vi "Main.vi"() -> ()   [LabVIEW 2020]
uses:
  Global Variables/Global Number of Indices.vi
  Global Variables/Training_Status.vi
  Global Variables/Number_of_Windows.vi
  Global Variables/Window_Size.vi
  Global Variables/Global Label.vi
  Global Variables/Global N-Back Setting.vi
  Global Variables/Trainning Done.vi
  Global Variables/Global Send To ANN.vi
  Global Variables/Global Difficulty Level.vi
  Global Variables/Global Enable Logging.vi
  Global Variables/Global User_Answer.vi
  Global Variables/Global Correct Answer.vi
panel:
  out "Difficulty Level":u8
  out "tiggerTime":u32
  out "New square":T1
  out "seq":i8
  out "Data":bool[](array[boolean])
  out "error out":errorcluster
  out "2D Picture":picture
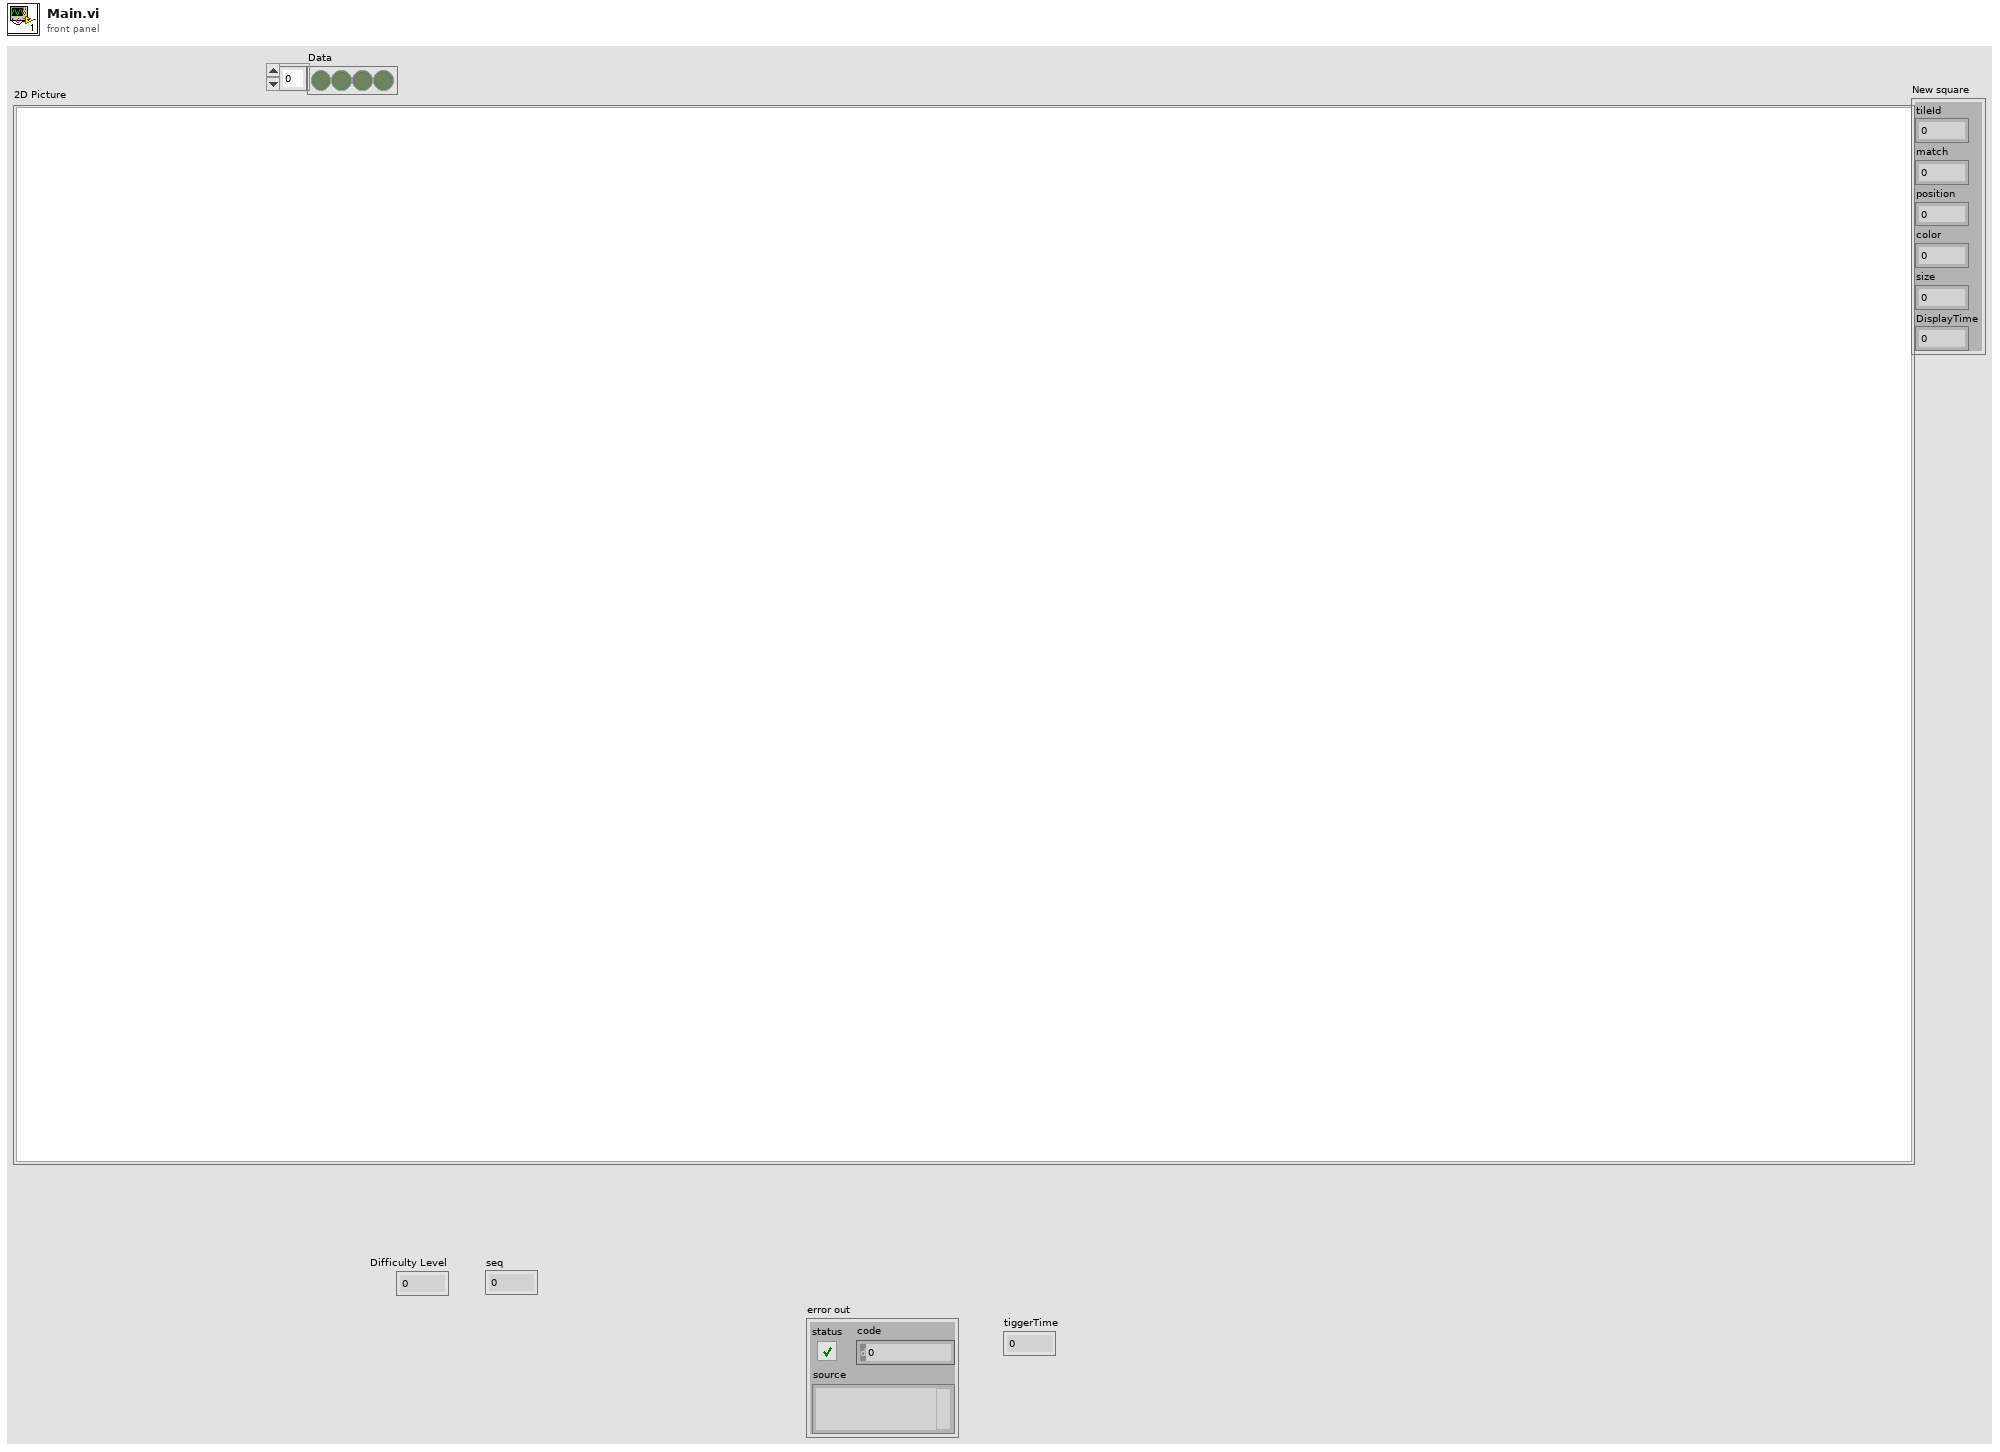
[diagram p1: front panel]
types:
  T1 = cluster{"tileId":i32, "match":i32, "position":i32, "color":u32, "size":i32, "DisplayTime":i32}
  T2 = cluster{"State":i32, "Iteration":i8, "Sequence":i8, "Counter":i8}
  T3 = cluster{"Tile size Y":dbl, "Columns":dbl, "Rows":dbl, "Cross size":dbl, "Offset X":dbl, "Tile size X":dbl, "OffsetY":dbl}
  T4 = cluster{"tileId":i32, "match":i32, "position":i32, "color":u32, "size":i32, "DisplayTime":i32}[]
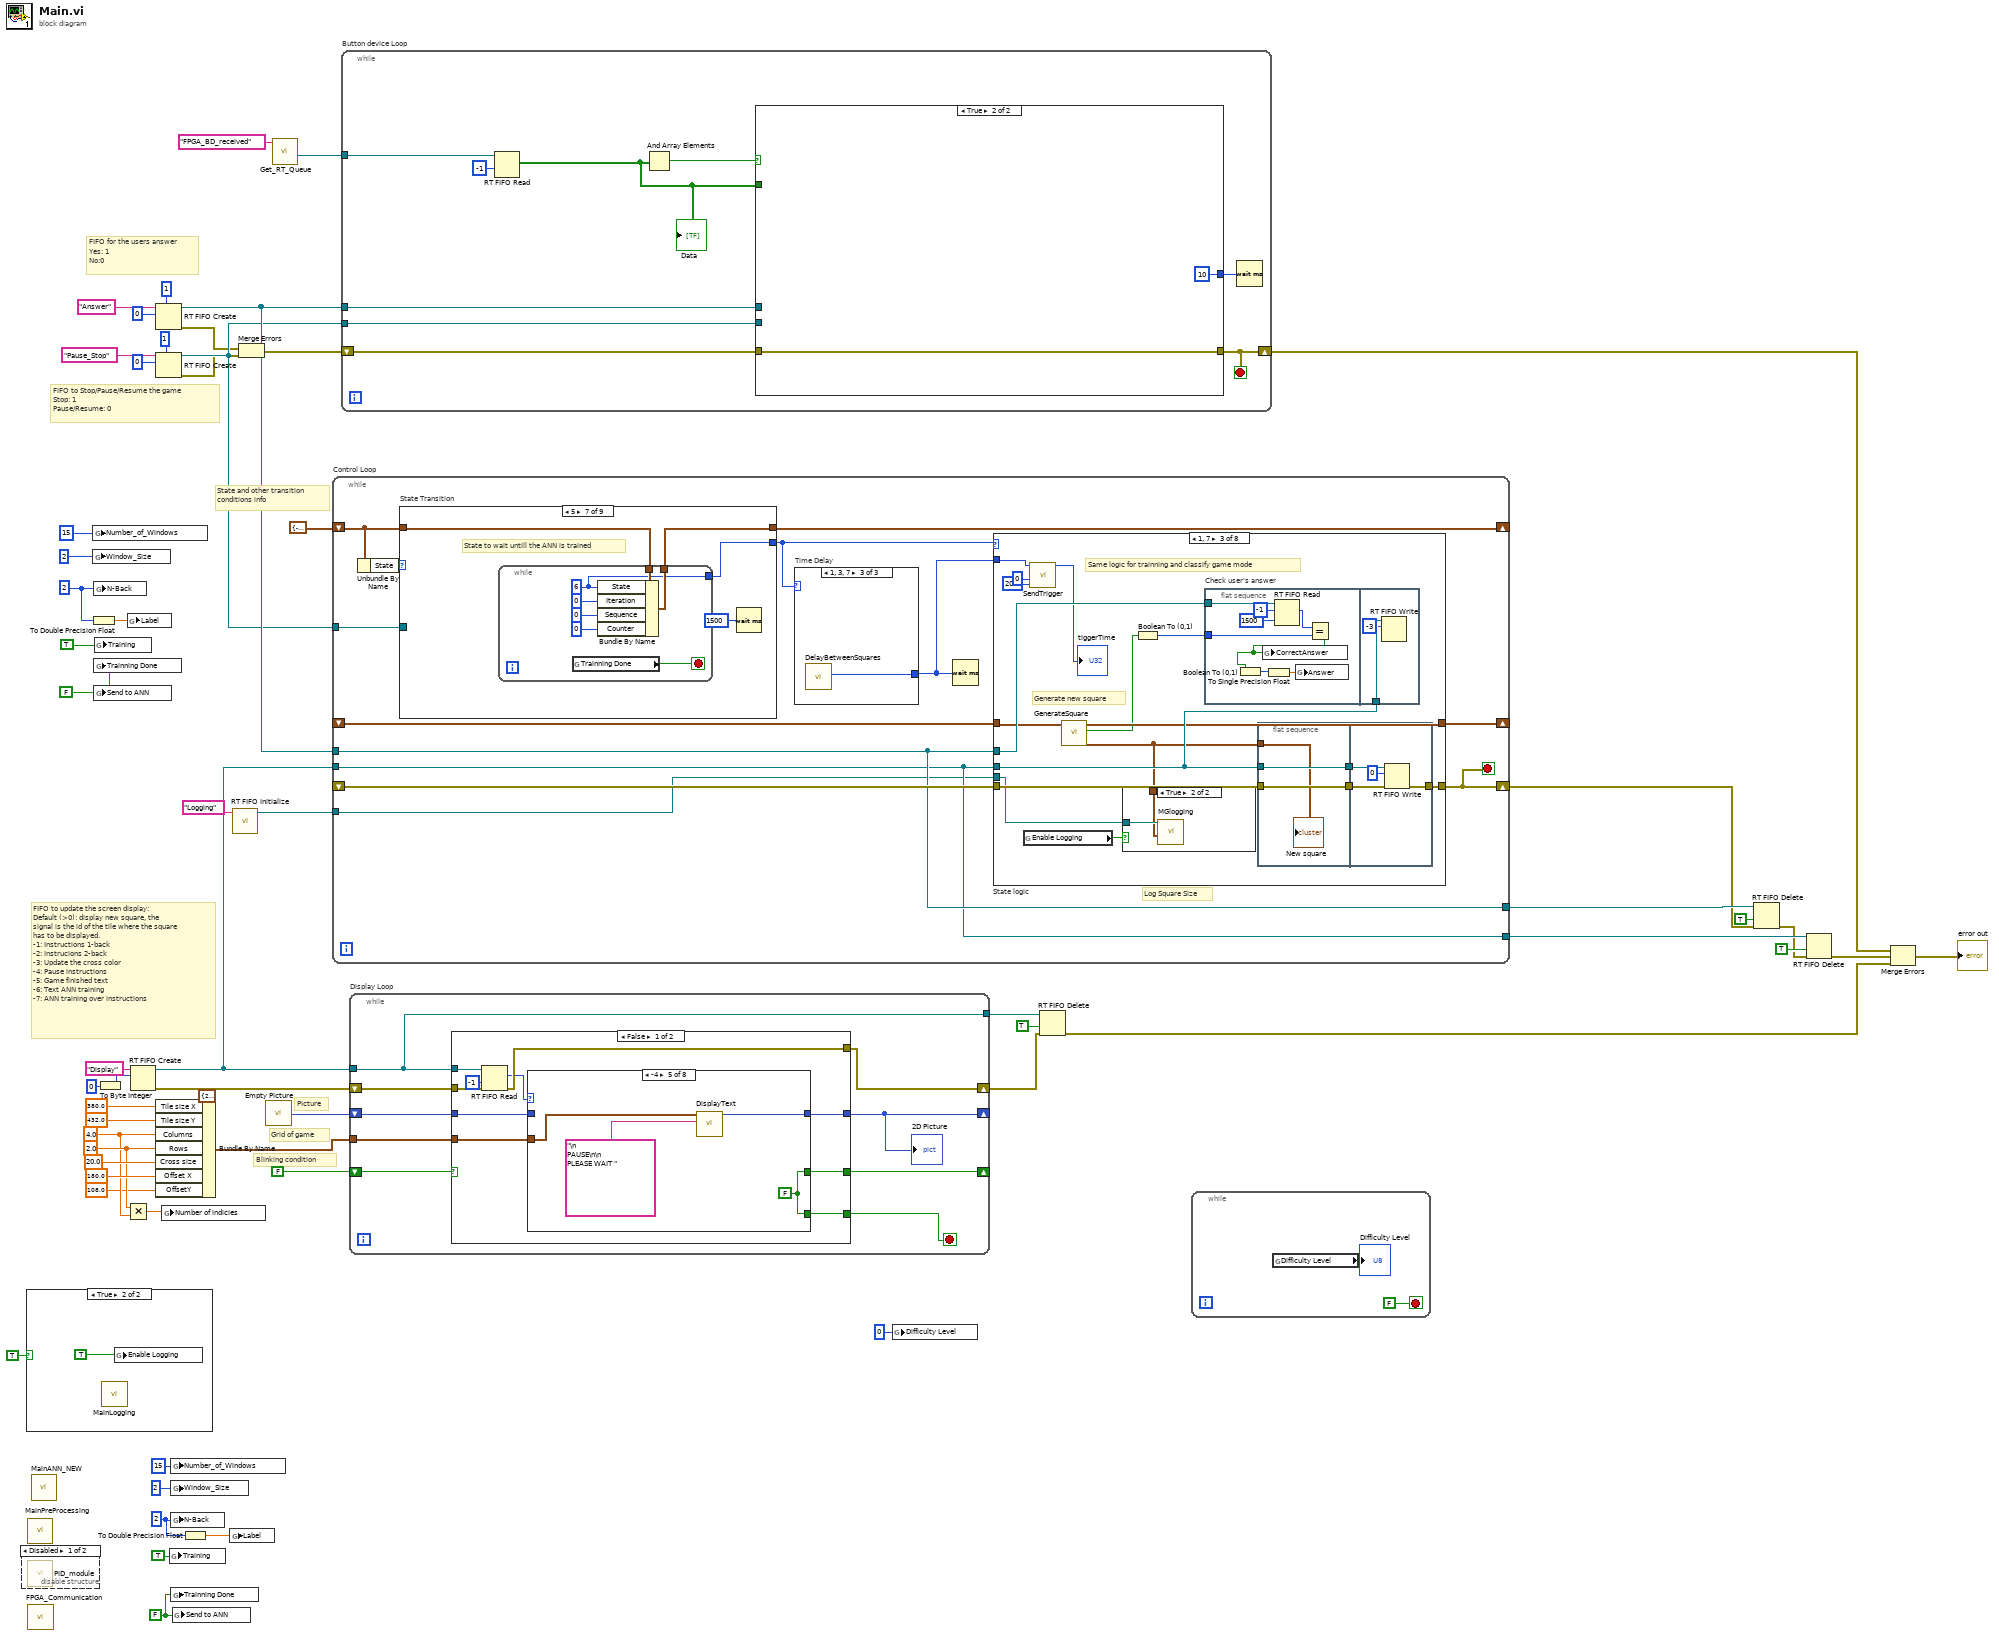
[diagram p0: block diagram]
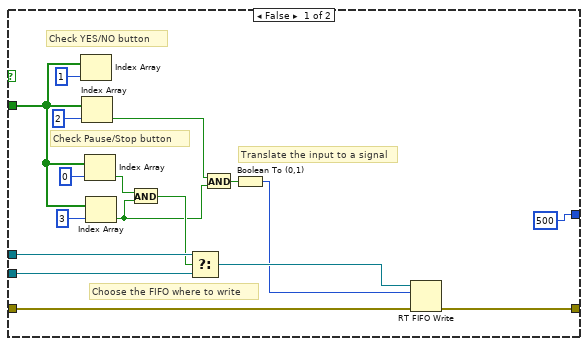
[diagram p3: hidden frame]
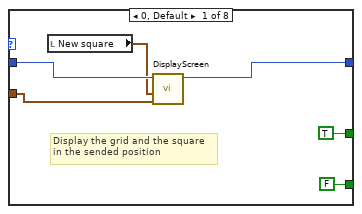
[diagram p5: hidden frame]
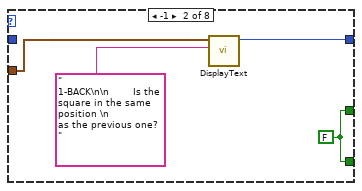
[diagram p6: hidden frame]
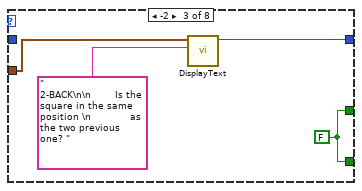
[diagram p7: hidden frame]
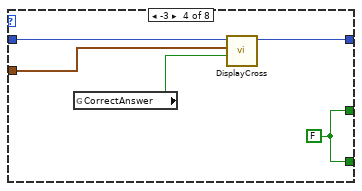
[diagram p8: hidden frame]
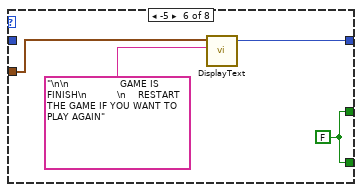
[diagram p9: hidden frame]
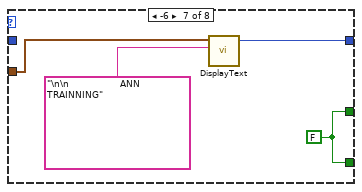
[diagram p10: hidden frame]
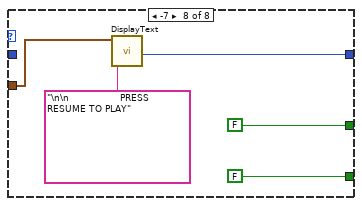
[diagram p11: hidden frame]
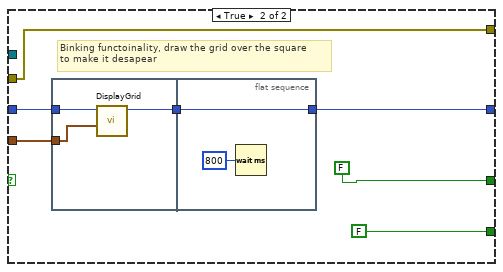
[diagram p12: hidden frame]
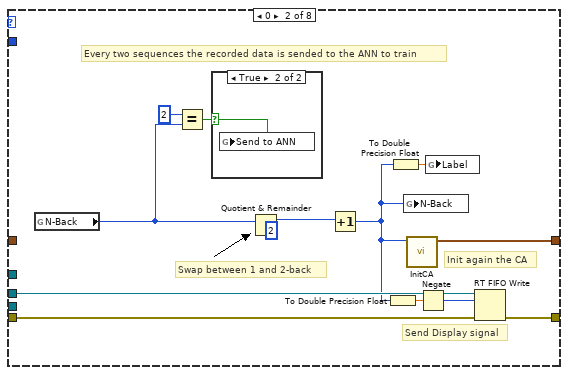
[diagram p14: hidden frame]
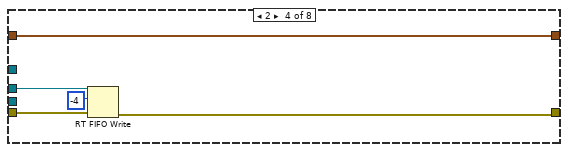
[diagram p17: hidden frame]
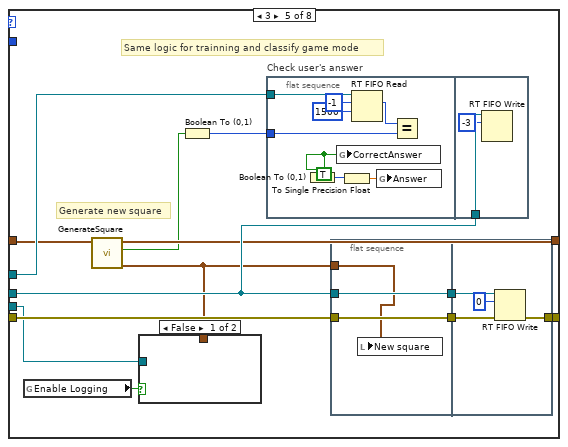
[diagram p18: hidden frame]
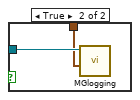
[diagram p19: hidden frame]
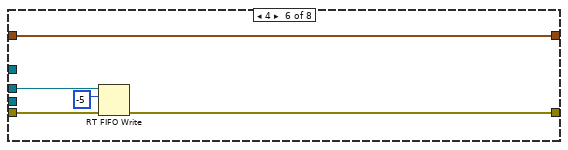
[diagram p20: hidden frame]
diagram:
  w5 = FALSE ("Send to ANN")
  w6 = u8 2 ("N-Back")
  w16 = FALSE ("Send to ANN")
  w17 = u8 2 ("N-Back")
  w47 = 2.0 ("Rows")
  w46 = 4.0 ("Columns")
  # "State and other transition \nconditions info"
  # "Picture"
  # "Grid of game"
  # "Blinking condition"
  # "FIFO to update the screen display:\nDefault (>0): display new square, the \nsignal is the id of the tile where the square\nhas to be displayed.\n-1: Instructions 1-back \n-2: Instrucions 2-back\n-3: Update the cross color \n-4: Pause instructions \n-5: Game finished text\n-6: Text ANN training\n-7: ANN training over instructions"
  # "FIFO to Stop/Pause/Resume the game\nStop: 1\nPause/Resume: 0"
  # "FIFO for the users answer\nYes: 1\nNo:0"
  n1 = disable-structure shown="Disabled" {
    frame Disabled {
      n2 = call "PID_module.vi"() -> ()  [unwired: 11 in]
    }
    frame Enabled {
    }
  }
  n3 = case shown="True" TRUE {
    frame False {
    }
    frame True {
      n4 = call "MainLogging.vi"() -> ()  [unwired: 7 in]
      n5 = global write "Global Enable Logging.vi" "Enable Logging"(TRUE ("Enable Logging")) -> ()
    }
  }
  n6 = call "MainPreProcessing.vi"() -> ()  [unwired: 12 in]
  n7 = call "FPGA_Communication.vi"() -> ()  [unwired: 12 in]
  n8 = call "MainANN_NEW.vi"() -> ()  [unwired: 12 in]
  n9 = To Double Precision Float(number=w17) -> (double precision float=w18:dbl)
  n10 = global write "Number_of_Windows.vi" "Number_of_Windows"(u32 15 ("Number of Windows")) -> ()
  n11 = global write "Window_Size.vi" "Window_Size"(u32 2 ("Window_Size")) -> ()
  n12 = global write "Global N-Back Setting.vi" "N-Back"(w17) -> ()
  n13 = global write "Trainning Done.vi" "Trainning Done"(w16) -> ()
  n14 = global write "Global Send To ANN.vi" "Send to ANN"(w16) -> ()
  n15 = global write "Training_Status.vi" "Training"(TRUE ("Training")) -> ()
  n16 = To Byte Integer(number=0) -> (8bit integer=w57:i8)
  n17 = Multiply(x=w47, y=w46) -> (x*y=w48:dbl)
  n18 = global write "Global Label.vi" "Label"(w18) -> ()
  n19 = RT FIFO Create(0:"Display" ("name (unnamed)"), 1:w57) -> (8:w55:refnum<k33>, 11:w36:errorcluster)  [unwired: 6 in, 1 out]
  n20 = Bundle By Name(cluster=T3 {"Tile size Y"=250.0, "Columns"=4.0, "Rows"=2.0, "Cross size"=20.0, "Offset X"=98.0, "Tile size X"=250.0, "OffsetY"=98.0} ("Grid"), "Tile size X"=380.0, "Tile size Y"=432.0 ("Tile size"), "Columns"=w46, "Rows"=w47, "Cross size"=20.0, "Offset X"=180.0 ("Offset"), "OffsetY"=108.0) -> (w35:T3)
  n21 = RT FIFO Create(0:"Answer" ("name (unnamed)"), 1:i16 0, 4:u32 1 ("size (10)")) -> (8:w45:refnum<k33>, 11:w40:errorcluster)  [unwired: 5 in, 1 out]
  n22 = RT FIFO Create(0:"Pause_Stop" ("name (unnamed)"), 1:i16 0, 4:u32 1 ("size (10)")) -> (8:w44:refnum<k33>, 11:w39:errorcluster)  [unwired: 5 in, 1 out]
  n23 = global write "Global Number of Indices.vi" "Number of indicies"(w48) -> ()
  n24 = global write "Training_Status.vi" "Training"(TRUE ("Training")) -> ()
  n25 = global write "Number_of_Windows.vi" "Number_of_Windows"(u32 15 ("Number of Windows")) -> ()
  n26 = global write "Window_Size.vi" "Window_Size"(u32 2 ("Window_Size")) -> ()
  n27 = global write "Global N-Back Setting.vi" "N-Back"(w6) -> ()
  n28 = global write "Trainning Done.vi" "Trainning Done"(w5) -> ()
  n29 = global write "Global Send To ANN.vi" "Send to ANN"(w5) -> ()
  n30 = To Double Precision Float(number=w6) -> (double precision float=w7:dbl)
  n31 = global write "Global Label.vi" "Label"(w7) -> ()
  n32 = call "RT FIFO Initialize.vi"("name (unnamed)"="Logging") -> ("rt fifo"=w12:refnum<k33>)  [unwired: 9 in, 1 out]
  n33 = Merge Errors(w40, w39) -> (w38:errorcluster)
  n34 = call "Empty Picture"() -> ("empty picture"=w53:picture)
  n35 = call "Get_RT_Queue.vi"("String"="FPGA_BD_received") -> ("rt fifo boolean"=w3:refnum<k33>)  [unwired: 8 in, 2 out]
  n36 = while "Control Loop" {
    tunnel: w55 -> [w64]
    tunnel: w45 -> [w65]
    tunnel: w44 -> [w71]
    shift-right: [w72] -> _
    shift-left: T2 {"State"=-1, "Iteration"=0, "Sequence"=0, "Counter"=0} -> [w73]
    shift-right: [w63] -> _
    shift-left: _ -> [w69]
    shift-right: [w66] -> w31
    shift-left: _ -> [w68]
    tunnel: [w65] -> w33
    tunnel: [w64] -> w32
    tunnel: w12 -> [w62]
    stop <- w66 stop-if-true
    # "Log Square Size"
    n37 = Unbundle By Name(w73) -> ("State"=w74:i32)
    n38 = case "State Transition" shown="5" w74 {
      tunnel: w73 -> [w192 w202 w211 w231 w246 w254 w269 w286 w297]
      tunnel: [w191 w197 w212 w230 w244 w255 w270 w285 w296] -> w72
      tunnel: w71 -> [_ _ _ w229 w242 w253 _ w287 w295]
      tunnel: [w190 0 ("f") w203 w214 w243 w250 w268 w284 w288] -> w70
      frame Default {
        w190 = -4 ("State")
        n39 = Bundle By Name(cluster=w192, "State"=w190, "Iteration"=i8 0, "Sequence"=i8 0, "Counter"=i8 0) -> (w191:T2)
      }
      frame -1 {
        # "Start state"
        n40 = Bundle By Name(cluster=w202, "State"=0, "Iteration"=i8 -1, "Sequence"=i8 0, "Counter"=i8 0) -> (w197:T2)
      }
      frame 0 {
        # "Start sequence"
        # "Number of sequences to train the ANN"
        n41 = Unbundle By Name(w211) -> ("Sequence"=w210:i8)
        n42 = Increment(x=w210) -> (x+1=w205:i8)
        "seq" <- w205
        n43 = Less?(x=w205, y=i8 3) -> (x < y?=w208:bool)
        n44 = Select(t=3 ("State"), s=w208, f=5) -> (s? t:f=w203:i32)
        n45 = Bundle By Name(cluster=w211, "State"=w203, "Iteration"=i8 0 ("Sequence"), "Sequence"=w205, "Counter"=i8 0) -> (w212:T2)
      }
      frame 1 {
        # "Check for Pause signal"
        # "Increase iteration number"
        # "Playing in trainning mode"
        n46 = Unbundle By Name(w231) -> ("Iteration"=w236:i8, "Sequence"=w221:i8)
        n47 = RT FIFO Read(0:w229, 1:i8 -1 ("element")) -> (9:w227:i16)  [unwired: 2 in, 4 out]
        n48 = Increment(x=w236) -> (x+1=w234:i8)
        n49 = Equal?(x=w227, y=i8 0) -> (x = y?=w224:bool)
        n50 = Less?(x=w234, y=i8 7) -> (x < y?=w223:bool)
        n51 = Select(t=1 ("State"), s=w223, f=0) -> (s? t:f=w222:i32)
        n52 = Equal?(x=w221, y=i8 2) -> (x = y?=w218:bool)
        n53 = Select(t=2, s=w224, f=w222) -> (s? t:f=w215:i32)
        n54 = Equal To 0?(x=w222) -> (x = 0?=w219:bool)
        n55 = And(x=w218, y=w219) -> (x .and. y?=w217:bool)
        n56 = Select(t=5, s=w217, f=w215) -> (s? t:f=w214:i32)
        n57 = Bundle By Name(cluster=w231, "State"=w214, "Iteration"=w234, "Sequence"=w221, "Counter"=i8 0) -> (w230:T2)
      }
      frame 2 {
        # "Waits untill it gets a Stop/Pause signal"
        # "Pause State"
        n58 = global read "Trainning Done.vi" "Trainning Done"() -> (w241:bool)
        n59 = RT FIFO Read(0:w242, 2:-1 ("timeout in ms (0)")) -> (9:w248:i16)  [unwired: 2 in, 4 out]
        n60 = Equal To 0?(x=w248) -> (x = 0?=w247:bool)
        n61 = Select(t=7, s=w241, f=3 ("timeout in ms (0)")) -> (s? t:f=w238:i32)
        n62 = Select(t=w238, s=w247, f=4) -> (s? t:f=w243:i32)
        n63 = Bundle By Name(cluster=w246, "State"=w243) -> (w244:T2)
      }
      frame 3 {
        # "State: back to normal"
        n64 = Unbundle By Name(w254) -> ("Sequence"=w262:i8, "Counter"=w252:i8)
        n65 = RT FIFO Read(0:w253, 1:i8 -1 ("element")) -> (9:w260:i16)  [unwired: 2 in, 4 out]
        n66 = Increment(x=w252) -> (x+1=w251:i8)
        n67 = Equal?(x=w260, y=i8 1) -> (x = y?=w258:bool)
        n68 = Less?(x=w251, y=i8 3) -> (x < y?=w265:bool)
        n69 = Select(t=3 ("State"), s=w265, f=1) -> (s? t:f=w257:i32)
        n70 = Select(t=2, s=w258, f=w257) -> (s? t:f=w250:i32)
        n71 = Bundle By Name(cluster=w254, "State"=w250, "Sequence"=w262, "Counter"=w251) -> (w255:T2)
      }
      frame 5 {
        # "State to wait untill the ANN is trained"
        n72 = while {
          tunnel: [w273] -> w270
          tunnel: w269 -> [w272]
          tunnel: [w271] -> w268
          stop <- w277 stop-if-true
          w271 = 6 ("State")
          n73 = global read "Trainning Done.vi" "Trainning Done"() -> (w277:bool)
          n74 = Bundle By Name(cluster=w272, "State"=w271, "Iteration"=i8 0, "Sequence"=i8 0, "Counter"=i8 0) -> (w273:T2)
        }
        n75 = Wait (ms)(milliseconds to wait=u32 1500) -> ()  [unwired: 1 out]
      }
      frame 6 {
        w284 = 7 ("s? t:f")
        # "State to wait to start to play classify"
        n76 = RT FIFO Read(0:w287, 2:-1 ("timeout in ms (0)")) -> (9:w282:i16)  [unwired: 2 in, 4 out]
        n77 = global write "Global Difficulty Level.vi" "Difficulty Level"(u8 1 ("Difficulty Level")) -> ()
        n78 = Equal To 0?(x=w282) -> (x = 0?=w281:bool)
        n79 = Select(t=7 ("timeout in ms (0)"), s=w281, f=4) -> ()  [unwired: 1 out]
        n80 = Bundle By Name(cluster=w286, "State"=w284) -> (w285:T2)
      }
      frame 7 {
        # "Check for pause signal"
        # "Playing classification"
        n81 = RT FIFO Read(0:w295, 1:i8 -1 ("element")) -> (9:w293:i16)  [unwired: 2 in, 4 out]
        n82 = Equal?(x=w293, y=i8 0) -> (x = y?=w291:bool)
        n83 = Select(t=2, s=w291, f=7) -> (s? t:f=w288:i32)
        n84 = Bundle By Name(cluster=w297, "State"=w288, "Counter"=i8 0) -> (w296:T2)
      }
    }
    n85 = case "Time Delay" shown="1, 3, 7" w70 {
      tunnel: [0 ("f") i64 6000 ("f") w189] -> w67
      frame Default {
      }
      frame 0 {
        # "The instructions/Text\nis displaed for 4 s"
      }
      frame 1, 3, 7 {
        n86 = call "DelayBetweenSquares.vi"() -> ("milliseconds to wait"=w189:u32)  [unwired: 10 in]
      }
    }
    n87 = Wait (ms)(milliseconds to wait=w67) -> ()  [unwired: 1 out]
    n88 = case "State logic" shown="1, 7" w70 {
      tunnel: w64 -> [_ w87 w103 w131 w140 w167 w174 w184]
      tunnel: w65 -> [_ _ w105 _ w142 _ _ _]
      tunnel: w69 -> [w75 _ w101 w127 w138 w164 w169 _]
      tunnel: w68 -> [w76 w84 w106 w130 w143 w166 w173 w185]
      tunnel: [w76 w83 w107 w129 w144 w165 w172 w183] -> w66
      tunnel: w67 -> [_ _ w97 _ _ _ _ _]
      tunnel: [w75 w77 w102 w127 w139 w164 w169 w181] -> w63
      tunnel: w62 -> [_ _ w94 _ w134 _ _ _]
      frame Default {
      }
      frame 0 {
        # "Send Display signal"
        # "Init again the CA"
        # "Swap between 1 and 2-back"
        # "Every two sequences the recorded data is sended to the ANN to train"
        n89 = global read "Global N-Back Setting.vi" "N-Back"() -> (w79:u8)
        n90 = Equal?(x=u8 2, y=w79) -> (x = y?=w80:bool)
        n91 = case shown="True" w80 {
          selector: w80 -> [_ w90]
          frame False {
          }
          frame True {
            n92 = global write "Global Send To ANN.vi" "Send to ANN"(w90) -> ()
          }
        }
        n93 = Quotient & Remainder(x=w79, y=u8 2) -> (x-y*floor(x/y)=w88:u8)  [unwired: 1 out]
        n94 = Increment(x=w88) -> (x+1=w81:u8)
        n95 = To Double Precision Float(number=w81) -> (double precision float=w85:dbl)
        n96 = To Double Precision Float(number=w81) -> (double precision float=w82:dbl)
        n97 = global write "Global N-Back Setting.vi" "N-Back"(w81) -> ()
        n98 = call "InitCA.vi"("N-Back"=w81) -> ("CA"=w77:T4)  [unwired: 10 in]
        n99 = Negate(x=w85) -> (-x=w86:i8)
        n100 = global write "Global Label.vi" "Label"(w82) -> ()
        n101 = RT FIFO Write(0:w87, 1:w86, 3:w84) -> (11:w83:errorcluster)  [unwired: 2 in, 3 out]
      }
      frame 1, 7 {
        # "Same logic for trainning and classify game mode"
        # "Generate new square"
        n102 = global read "Global Enable Logging.vi" "Enable Logging"() -> (w92:bool)
        n103 = call "SendTrigger.vi"("System Exe time"=200, "Window time"=0, "TimeSquares"=w97) -> ("millisecond timer value"=→"tiggerTime":u32)  [unwired: 8 in]
        n104 = call "GenerateSquare.vi"("CA"=w101) -> ("New square"=w93:T1, "Match"=w98:bool, "updated CA"=w102:T4)  [unwired: 8 in]
        n105 = case shown="True" w92 {
          tunnel: w94 -> [_ w109]
          tunnel: w93 -> [_ w108]
          frame False {
          }
          frame True {
            n106 = call "MGlogging.vi"("New square"=w108, "Refnum in"=w109) -> ()  [unwired: 9 in, 1 out]
          }
        }
        n107 = Boolean To (0,1)(Boolean=w98) -> (0, 1=w104:i16)
        n108 = flat-sequence "Check user's answer" {
          tunnel: w105 -> [w124]
          tunnel: w104 -> [w120]
          tunnel: w103 -> [w126]
          frame #0 {
            n109 = RT FIFO Read(0:w124, 1:i16 -1 ("element"), 2:1500 ("timeout in ms (0)")) -> (9:w121:i16)  [unwired: 1 in, 4 out]
            n110 = Equal?(x=w121, y=w120) -> (x = y?=w117:bool)
            n111 = Boolean To (0,1)(Boolean=w117) -> (0, 1=w119:i16)
            n112 = global write "Global Correct Answer.vi" "CorrectAnswer"(w117) -> ()
            n113 = To Single Precision Float(number=w119) -> (single precision float=w118:sgl)
            n114 = global write "Global User_Answer.vi" "Answer"(w118) -> ()
          }
          frame #1 {
            n115 = RT FIFO Write(0:w126, 1:i8 -3 ("element")) -> ()  [unwired: 3 in, 4 out]
          }
        }
        n116 = flat-sequence {
          tunnel: w103 -> [w111]
          tunnel: w106 -> [w112]
          tunnel: [w112] -> w100
          tunnel: [w111] -> w99
          tunnel: w93 -> [w110]
          tunnel: [w116] -> w107
          tunnel: w100 -> [w115]
          tunnel: w99 -> [w114]
          frame #0 {
            "New square" <- w110
          }
          frame #1 {
            n117 = RT FIFO Write(0:w114, 1:i8 0 ("element"), 3:w115) -> (11:w116:errorcluster)  [unwired: 2 in, 3 out]
          }
        }
      }
      frame 2 {
        n118 = RT FIFO Write(0:w131, 1:i8 -4 ("element"), 3:w130) -> (11:w129:errorcluster)  [unwired: 2 in, 3 out]
      }
      frame 3 {
        # "Same logic for trainning and classify game mode"
        # "Generate new square"
        n119 = global read "Global Enable Logging.vi" "Enable Logging"() -> (w132:bool)
        n120 = call "GenerateSquare.vi"("CA"=w138) -> ("New square"=w133:T1, "Match"=w135:bool, "updated CA"=w139:T4)  [unwired: 8 in]
        n121 = case shown="False" w132 {
          tunnel: w134 -> [_ w146]
          tunnel: w133 -> [_ w145]
          frame False {
          }
          frame True {
            n122 = call "MGlogging.vi"("New square"=w145, "Refnum in"=w146) -> ()  [unwired: 9 in, 1 out]
          }
        }
        n123 = Boolean To (0,1)(Boolean=w135) -> (0, 1=w141:i16)
        n124 = flat-sequence "Check user's answer" {
          tunnel: w142 -> [w161]
          tunnel: w141 -> [w157]
          tunnel: w140 -> [w163]
          frame #0 {
            w154 = TRUE ("CorrectAnswer")
            n125 = Boolean To (0,1)(Boolean=w154) -> (0, 1=w156:i16)
            n126 = global write "Global Correct Answer.vi" "CorrectAnswer"(w154) -> ()
            n127 = To Single Precision Float(number=w156) -> (single precision float=w155:sgl)
            n128 = RT FIFO Read(0:w161, 1:i16 -1 ("element"), 2:1500 ("timeout in ms (0)")) -> (9:w158:i16)  [unwired: 1 in, 4 out]
            n129 = global write "Global User_Answer.vi" "Answer"(w155) -> ()
            n130 = Equal?(x=w158, y=w157) -> ()  [unwired: 1 out]
          }
          frame #1 {
            n131 = RT FIFO Write(0:w163, 1:i8 -3 ("element")) -> ()  [unwired: 3 in, 4 out]
          }
        }
        n132 = flat-sequence {
          tunnel: w140 -> [w148]
          tunnel: w143 -> [w149]
          tunnel: [w149] -> w137
          tunnel: [w148] -> w136
          tunnel: w133 -> [w147]
          tunnel: [w153] -> w144
          tunnel: w137 -> [w152]
          tunnel: w136 -> [w151]
          frame #0 {
            n133 = local write "New square"(w147) -> ()
          }
          frame #1 {
            n134 = RT FIFO Write(0:w151, 1:i8 0 ("element"), 3:w152) -> (11:w153:errorcluster)  [unwired: 2 in, 3 out]
          }
        }
      }
      frame 4 {
        n135 = RT FIFO Write(0:w167, 1:i8 -5 ("element"), 3:w166) -> (11:w165:errorcluster)  [unwired: 2 in, 3 out]
      }
      frame 5 {
        w170 = u8 2 ("N-Back")
        n136 = flat-sequence {
          frame #0 {
            n137 = global write "Global Send To ANN.vi" "Send to ANN"(TRUE ("Send to ANN")) -> ()
          }
          frame #1 {
            n138 = global write "Training_Status.vi" "Training"(FALSE ("Training")) -> ()
          }
          frame #2 {
            n139 = call "SendTrigger.vi"("System Exe time"=200, "Window time"=40, "TimeSquares"=1000) -> ()  [unwired: 8 in, 1 out]
          }
        }
        n140 = global write "Global N-Back Setting.vi" "N-Back"(w170) -> ()
        n141 = To Double Precision Float(number=w170) -> (double precision float=w171:dbl)
        n142 = global write "Global Label.vi" "Label"(w171) -> ()
        n143 = RT FIFO Write(0:w174, 1:i8 -6 ("element"), 3:w173) -> (11:w172:errorcluster)  [unwired: 2 in, 3 out]
      }
      frame 6 {
        # "Init the CA for the classify mode"
        n144 = global read "Global N-Back Setting.vi" "N-Back"() -> (w182:u8)
        n145 = RT FIFO Write(0:w184, 1:i8 -7 ("element"), 3:w185) -> (11:w183:errorcluster)  [unwired: 2 in, 3 out]
        n146 = call "InitCA.vi"("N-Back"=w182) -> ("CA"=w181:T4)  [unwired: 10 in]
      }
    }
  }
  n147 = while "Button device Loop" {
    tunnel: w45 -> [w307]
    tunnel: w44 -> [w306]
    shift-right: [w304] -> w27
    shift-left: w38 -> [w305]
    tunnel: w3 -> [w302]
    stop <- w304 stop-if-true
    n148 = RT FIFO Read(0:w302, 2:-1 ("timeout in ms (0)")) -> (9:w300:bool[])  [unwired: 2 in, 4 out]
    "Data" <- w300
    n149 = And Array Elements(Boolean array=w300) -> (logical AND=w303:bool)
    n150 = case shown="True" w303 {
      tunnel: w300 -> [w318 _]
      tunnel: w307 -> [w324 _]
      tunnel: w306 -> [w323 _]
      tunnel: w305 -> [w312 w326]
      tunnel: [w311 w326] -> w304
      tunnel: [500 ("index") 10 ("index")] -> w299
      frame False {
        # "Translate the input to a signal"
        # "Choose the FIFO where to write"
        # "Check Pause/Stop button"
        # "Check YES/NO button"
        n151 = Index Array(array=w318, index=1) -> ()  [unwired: 1 out]
        n152 = Index Array(array=w318, index=2) -> (element=w316:bool)
        n153 = Index Array(array=w318, index=0) -> (element=w310:bool)
        n154 = Index Array(array=w318, index=3) -> (element=w309:bool)
        n155 = And(x=w310, y=w309) -> (x .and. y?=w317:bool)
        n156 = Select(t=w324, s=w317, f=w323) -> (s? t:f=w314:refnum<k33>)
        n157 = And(x=w316, y=w309) -> (x .and. y?=w315:bool)
        n158 = Boolean To (0,1)(Boolean=w315) -> (0, 1=w313:i16)
        n159 = RT FIFO Write(0:w314, 1:w313, 3:w312) -> (11:w311:errorcluster)  [unwired: 2 in, 3 out]
      }
      frame True {
      }
    }
    n160 = Wait (ms)(milliseconds to wait=w299) -> ()  [unwired: 1 out]
  }
  n161 = while "Display Loop" {
    tunnel: w55 -> [w329]
    shift-right: [w334] -> _
    shift-left: FALSE -> [w335]
    shift-right: [w332] -> _
    shift-left: w53 -> [w333]
    tunnel: w35 -> [w331]
    tunnel: [w329] -> w37
    shift-right: [w327] -> w15
    shift-left: w36 -> [w328]
    stop <- w330 stop-if-true
    n162 = case shown="False" w335 {
      tunnel: [w340 FALSE] -> w334
      tunnel: w333 -> [w343 w386]
      tunnel: [w341 w385] -> w332
      tunnel: w331 -> [w342 w384]
      tunnel: w329 -> [w345 _]
      tunnel: [w339 FALSE] -> w330
      tunnel: w328 -> [w338 w382]
      tunnel: [w337 w382] -> w327
      frame False {
        n163 = RT FIFO Read(0:w345, 2:-1 ("timeout in ms (0)"), 3:w338) -> (9:w336:i8, 11:w337:errorcluster)  [unwired: 1 in, 3 out]
        n164 = case shown="-4" w336 {
          tunnel: [TRUE w353 w357 w360 w365 w369 w373 FALSE] -> w340
          tunnel: [w348 w355 w356 w362 w366 w370 w374 w379] -> w341
          tunnel: w343 -> [w350 _ _ w363 _ _ _ _]
          tunnel: w342 -> [w347 w352 w359 w361 w367 w371 w375 w380]
          tunnel: [FALSE w353 w357 w360 w365 w369 w373 FALSE] -> w339
          frame 0, Default {
            # "Display the grid and the square\nin the sended position"
            n165 = local read "New square"() -> (w346:T1)
            n166 = call "DisplayScreen.vi"("Grid"=w347, "square"=w346, "input picture"=w350) -> ("2D Picture"=w348:picture)  [unwired: 8 in]
          }
          frame -1 {
            w353 = FALSE
            n167 = call "DisplayText.vi"("text"="                      1-BACK\n\n        Is the square in the same position \n                as the previous one? ", "Grid"=w352) -> ("new picture"=w355:picture)  [unwired: 9 in]
          }
          frame -2 {
            w357 = FALSE
            n168 = call "DisplayText.vi"("text"="                      2-BACK\n\n        Is the square in the same position \n             as the two previous one? ", "Grid"=w359) -> ("new picture"=w356:picture)  [unwired: 9 in]
          }
          frame -3 {
            w360 = FALSE
            n169 = global read "Global Correct Answer.vi" "CorrectAnswer"() -> (w364:bool)
            n170 = call "DisplayCross.vi"("CorrectAnswer"=w364, "Grid"=w361, "new picture in"=w363) -> ("new picture out"=w362:picture)  [unwired: 8 in]
          }
          frame -4 {
            w365 = FALSE
            n171 = call "DisplayText.vi"("text"="\n                              PAUSE\n\n                   PLEASE WAIT ", "Grid"=w367) -> ("new picture"=w366:picture)  [unwired: 9 in]
          }
          frame -5 {
            w369 = FALSE
            n172 = call "DisplayText.vi"("text"="\n\n                 GAME IS FINISH\n          \n    RESTART THE GAME IF YOU WANT TO PLAY AGAIN", "Grid"=w371) -> ("new picture"=w370:picture)  [unwired: 9 in]
          }
          frame -6 {
            w373 = FALSE
            n173 = call "DisplayText.vi"("text"="\n\n                 ANN TRAINNING", "Grid"=w375) -> ("new picture"=w374:picture)  [unwired: 9 in]
          }
          frame -7 {
            n174 = call "DisplayText.vi"("text"="\n\n                 PRESS RESUME TO PLAY", "Grid"=w380) -> ("new picture"=w379:picture)  [unwired: 9 in]
          }
        }
      }
      frame True {
        # "Binking functoinality, draw the grid over the square\nto make it desapear"
        n175 = flat-sequence {
          tunnel: [w391] -> w387
          tunnel: w386 -> [w390]
          tunnel: w384 -> [w389]
          tunnel: [w392] -> w385
          tunnel: w387 -> [w392]
          frame #0 {
            n176 = call "DisplayGrid.vi"("Grid"=w389, "input picture"=w390) -> ("new picture"=w391:picture)  [unwired: 9 in]
          }
          frame #1 {
            n177 = Wait (ms)(milliseconds to wait=u32 800) -> ()  [unwired: 1 out]
          }
        }
      }
    }
    "2D Picture" <- w332
  }
  n178 = global write "Global Difficulty Level.vi" "Difficulty Level"(u8 0 ("Difficulty Level")) -> ()
  n179 = RT FIFO Delete(0:w37, 2:TRUE ("force destroy? (F)"), 3:w15) -> (11:w25:errorcluster)
  n180 = while {
    stop <- FALSE stop-if-true
    n181 = global read "Global Difficulty Level.vi" "Difficulty Level"() -> (→"Difficulty Level":u8)
  }
  n182 = RT FIFO Delete(0:w33, 2:TRUE ("force destroy? (F)"), 3:w31) -> (11:w28:errorcluster)
  n183 = RT FIFO Delete(0:w32, 2:TRUE ("force destroy? (F)"), 3:w28) -> (11:w26:errorcluster)
  n184 = Merge Errors(w27, w26, w25) -> (→"error out":errorcluster)
